vi "Main Page.vi"(8 "error in (no error)":errorcluster, 11 "Node Ptr":T1 format="%.0x") -> (0 "error out":errorcluster)   [LabVIEW 2019, in "UDP-Custom-Device System Explorer.lvlib"]
uses:
  UDP-Custom-Device System Explorer.lvlib
  <vilib>/NI VeriStand/Custom Device API/Custom Device Item Ref.ctl
  Types/Page References/Refs - Main Page.ctl
  <vilib>/NI VeriStand/Custom Device API/Custom Device API.lvlib
  <vilib>/NI VeriStand/Custom Device Tools/Custom Device Utility Library/Custom Device Utility Library.lvlib
  Property Accessors/Main Accessors.lvlib
panel:
  in  "Export Path":path
  in  "Export to File on Save":bool
  in  "Export Configuration Header":cluster{"Section Name":string}={"Section Name"="UDP Export Configuration Settings"}
  in  "Select Time-Stamp Channel":bool
  out "Timestamp Channel":string
  out "Version":string
  in  "SHDocVw.IWebBrowser":refnum<k7>(container)
  in  "Network Settings Header":cluster{"Section Name":string}={"Section Name"="UDP Settings"}
  in  "General Header":cluster{"Section Name":string}={"Section Name"="UDP Custom Device Information"}
  in  "Description":string
  in  "Name":string
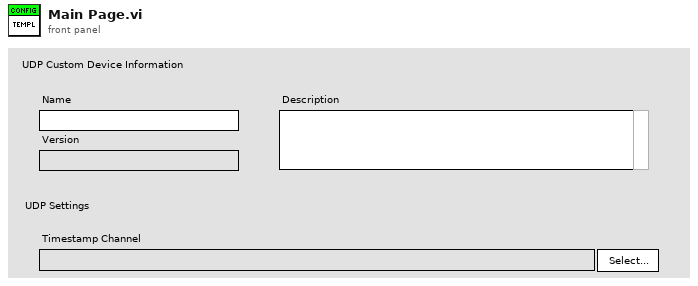
[diagram p1: front panel]
types:
  T1 = typedef "Custom Device API.lvlib/Custom Device Item Ref.ctl" = u64
  T2 = typedef "UDP-Custom-Device System Explorer.lvlib/Refs - Main Page.ctl" = cluster{"Name":refnum<vi>, "Timestamp Channel":refnum<vi>, "Export Path":refnum<vi>, "Export to File on Save":refnum<vi>}
  T3 = enum8{"Enabled", "Disabled", "Disabled and Grayed Out"}
  T4 = typedef "Custom Device API.lvlib/Custom Device Commands.ctl" = enum16{"Default", "Item renamed", "Shutdown", "Dynamic button pressed"}
  T5 = typedef "Custom Device API.lvlib/Custom Device Item Info.ctl" = cluster{"Name":string, "Is Channel":bool, "GUID":string, "Is Waveform":bool}
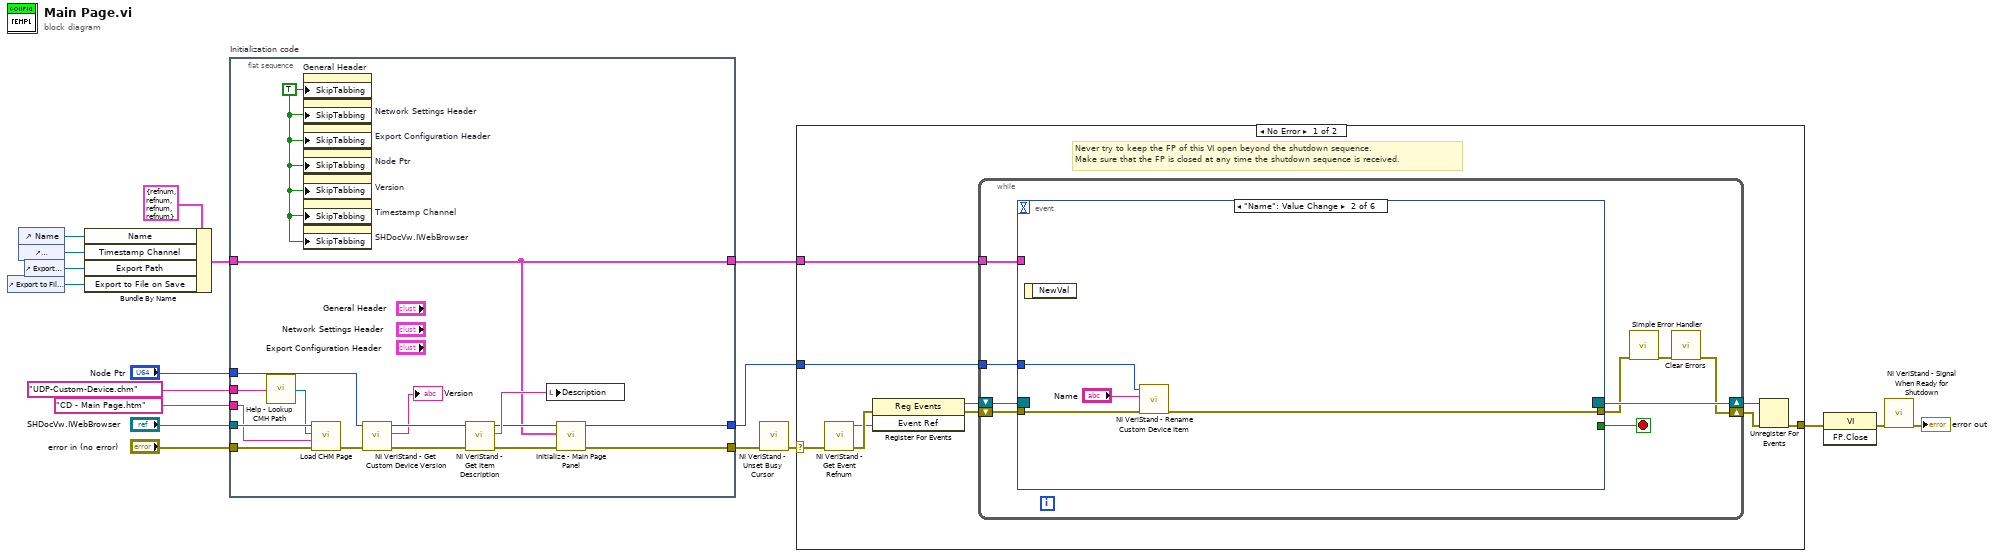
[diagram p0: block diagram]
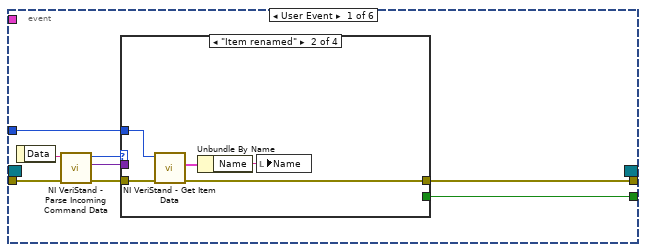
[diagram p2: hidden frame]
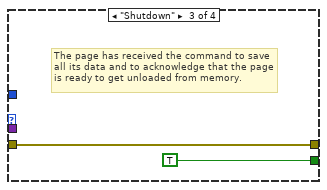
[diagram p4: hidden frame]
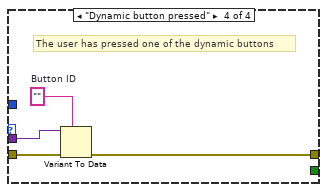
[diagram p5: hidden frame]
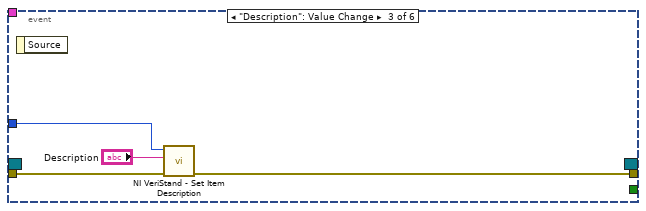
[diagram p6: hidden frame]
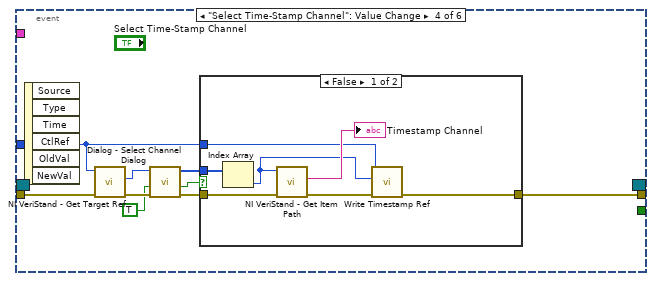
[diagram p7: hidden frame]
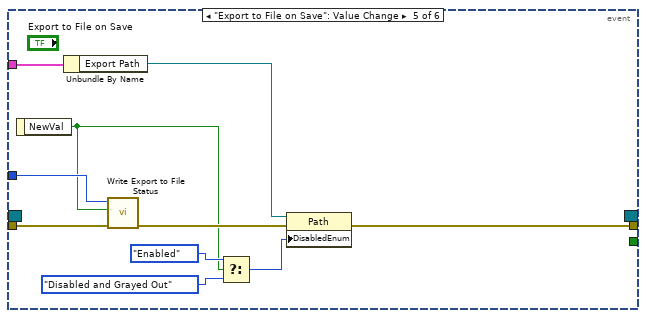
[diagram p9: hidden frame]
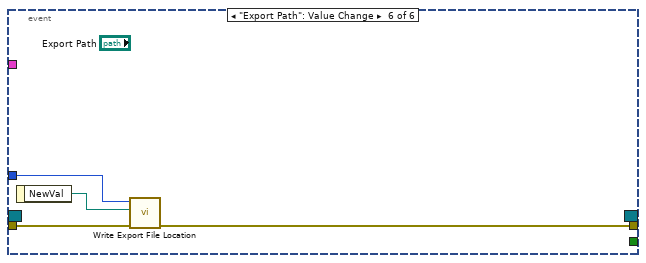
[diagram p10: hidden frame]
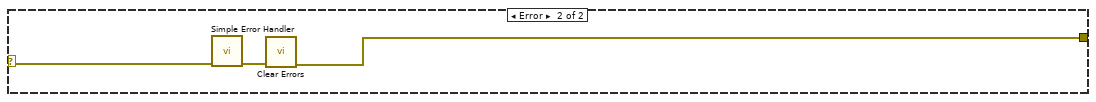
[diagram p11: hidden frame]
diagram:
  n1 = control-ref of="Export to File on Save"() -> (w4:refnum<vi>)
  n2 = control-ref of="Name"() -> (w1:refnum<vi>)
  n3 = control-ref of="Timestamp Channel"() -> (w6:refnum<vi>)
  n4 = control-ref of="Export Path"() -> (w5:refnum<vi>)
  n5 = Bundle By Name(cluster=T2 {"Name"=refnum, "Timestamp Channel"=refnum, "Export Path"=refnum, "Export to File on Save"=refnum} ("Main Page Refs"), "Name"=w1, "Timestamp Channel"=w6, "Export Path"=w5, "Export to File on Save"=w4) -> (w3:T2)
  n6 = flat-sequence "Initialization code" {
    tunnel: "error in (no error)" -> [w22]
    tunnel: "Node Ptr" -> [w35]
    tunnel: [w29] -> w14
    tunnel: [w28] -> w11
    tunnel: "SHDocVw.IWebBrowser" -> [w24]
    tunnel: "CD - Main Page.htm" ("HTML File") -> [w23]
    tunnel: "UDP-Custom-Device.chm" ("CD_CHM_FileName") -> [w21]
    tunnel: w3 -> [w26]
    tunnel: [w26] -> w2
    frame #0 {
      w19 = TRUE ("Skip When Tabbing")
      n7 = call "Help - Lookup CMH Path.vi"("Main CMH File"=w21) -> ("Compiled CMH Path"=w20:path)
      n8 = property on="General Header" class="Clust (strict)"("SkipTabbing"=w19) -> ()  [unwired: 2 in, 2 out]
      n9 = property on="Network Settings Header" class="Clust (strict)"("SkipTabbing"=w19) -> ()  [unwired: 2 in, 2 out]
      n10 = property on="Export Configuration Header" class="Clust (strict)"("SkipTabbing"=w19) -> ()  [unwired: 2 in, 2 out]
      n11 = property on="Node Ptr" class="DigNum (strict)"("SkipTabbing"=w19) -> ()  [unwired: 2 in, 2 out]
      n12 = property on="Version" class="Str"("SkipTabbing"=w19) -> ()  [unwired: 2 in, 2 out]
      n13 = property on="Timestamp Channel" class="Str"("SkipTabbing"=w19) -> ()  [unwired: 2 in, 2 out]
      n14 = property on="SHDocVw.IWebBrowser" class="AXCont"("SkipTabbing"=w19) -> ()  [unwired: 2 in, 2 out]
      n15 = call <vilib>:"Load CHM Page.vi"("error in (no error)"=w22, "HTML File"=w23, "Compiled CHM Path"=w20, "Web Browser Reference"=w24) -> ("error out"=w25:errorcluster)  [unwired: 7 in]
      n16 = call <vilib>:"NI VeriStand - Get Custom Device Version.vi"("error in (no error)"=w25, "Device Ref in"=w35) -> ("error out"=w34:errorcluster, "Value"=→"Version":string, "Device Ref out"=w33:T1)  [unwired: 7 in]
      n17 = call <vilib>:"NI VeriStand - Get Item Description.vi"("error in (no error)"=w34, "Item Ref in"=w33) -> ("error out"=w30:errorcluster, "Description"=w31:string, "Item Ref out"=w27:T1)  [unwired: 7 out]
      n18 = local write "Description"(w31) -> ()
      n19 = call "Initialize - Main Page Panel.vi"("error in (no error)"=w30, "Main Page References"=w26, "Item Ref in"=w27) -> ("error out"=w29:errorcluster, "Item Ref out"=w28:T1)  [unwired: 7 in]
    }
  }
  n20 = call <vilib>:"NI VeriStand - Unset Busy Cursor.vi"("error in (no error)"=w14) -> ("error out"=w13:errorcluster)  [unwired: 10 out]
  n21 = case shown="No Error" w13 {
    selector: w13 -> [w37 w116]
    tunnel: [w42 w114] -> w18
    tunnel: w11 -> [w38 _]
    tunnel: w2 -> [w36 _]
    frame No Error {
      # "Never try to keep the FP of this VI open beyond the shutdown sequence.\nMake sure that the FP is closed at any time the shutdown sequence is received."
      n22 = call <vilib>:"NI VeriStand - Get Event Refnum.vi"("error in (no error)"=w37) -> ("error out"=w45:errorcluster, "Event Ref"=w41:refnum<user-event>)  [unwired: 9 out]
      n23 = register-events(error in=w45, w41) -> (reference out=w39:refnum<event-registration>, error out=w40:errorcluster)  [unwired: 1 in]
      n24 = while {
        tunnel: w38 -> [w50]
        shift-right: [w47] -> w43
        shift-left: w40 -> [w53]
        shift-right: [w54] -> w44
        shift-left: w39 -> [w52]
        tunnel: w36 -> [w46]
        stop <- w51 stop-if-true
        n25 = event shown="[1] \"Name\": Value Change" {
          selector: w52 -> [_ _ _ _ _ _]
          dyn-events: [_ _ _ _ _ _] -> w54
          timeout: _ -> [_ _ _ _ _ _]
          tunnel: w53 -> [w62 w78 w81 w90 w102 w112]
          tunnel: [w58 _ _ _ _ _] -> w51
          tunnel: [w57 w77 w80 w91 w104 w111] -> w49
          tunnel: w50 -> [w56 w76 w82 w88 w103 w113]
          tunnel: w46 -> [_ _ _ _ w109 _]
          event User Event {
            n26 = event-data() -> ("Data"=w61:string)  [unwired: 1 out]
            n27 = call <vilib>:"NI VeriStand - Parse Incoming Command Data.vi"("error in (no error)"=w62, "Incoming data"=w61) -> ("error out"=w60:errorcluster, "Outgoing data"=w55:variant, "Action"=w59:T4)  [unwired: 7 out]
            n28 = case shown="\"Item renamed\"" w59 {
              tunnel: w60 -> [w63 w68 w69 w74]
              tunnel: [_ _ TRUE _] -> w58
              tunnel: [w63 w65 w69 w71] -> w57
              tunnel: w56 -> [_ w67 _ _]
              tunnel: w55 -> [_ _ _ w73]
              frame "Default", Default {
              }
              frame "Item renamed" {
                n29 = call <vilib>:"NI VeriStand - Get Item Data.vi"("error in (no error)"=w68, "Item Ref in"=w67) -> ("error out"=w65:errorcluster, "Item Info"=w66:T5)  [unwired: 8 out]
                n30 = Unbundle By Name(w66) -> ("Name"=w64:string)
                n31 = local write "Name"(w64) -> ()
              }
              frame "Shutdown" {
                # "The page has received the command to save all its data and to acknowledge that the page is ready to get unloaded from memory."
              }
              frame "Dynamic button pressed" {
                w72 = ""  # Button ID
                # "The user has pressed one of the dynamic buttons"
                n32 = Variant To Data(error in=w74, type=w72, Variant=w73) -> (error out=w71:errorcluster)  [unwired: 1 out]
              }
            }
          }
          event "Name": Value Change {
            n33 = event-data() -> ()  [unwired: 2 out]
            n34 = call <vilib>:"NI VeriStand - Rename Custom Device Item.vi"("error in (no error)"=w78, "New Name"="Name", "Item Ref in"=w76) -> ("error out"=w77:errorcluster)  [unwired: 1 in, 7 out]
          }
          event "Description": Value Change {
            n35 = event-data() -> ()  [unwired: 2 out]
            n36 = call <vilib>:"NI VeriStand - Set Item Description.vi"("error in (no error)"=w81, "Description"="Description", "Item Ref in"=w82) -> ("error out"=w80:errorcluster)  [unwired: 8 out]
          }
          event "Select Time-Stamp Channel": Value Change {
            n37 = event-data() -> ()  [unwired: 7 out]
            n38 = call <vilib>:"NI VeriStand - Get Target Ref.vi"("error in"=w90, "Item Ref in"=w88) -> ("error out"=w89:errorcluster, "Target Ref"=w87:T1)  [unwired: 6 in, 2 out]
            n39 = call "Dialog - Select Channel Dialog.vi"("error in (no error)"=w89, "Allow Section Selection (F)"=TRUE, "Root Item Ref"=w87) -> ("error out"=w85:errorcluster, "Canceled"=w83:bool, "Selected Channel Refs"=w84:T1[])  [unwired: 6 in]
            n40 = case shown="False" w83 {
              tunnel: [w92 w99] -> w91
              tunnel: w88 -> [w95 _]
              tunnel: w85 -> [w97 w99]
              tunnel: w84 -> [w98 _]
              frame False {
                n41 = Index Array(array=w98) -> (element=w94:T1)  [unwired: 1 in]
                n42 = call <vilib>:"NI VeriStand - Get Item Path.vi"("error in (no error)"=w97, "Item Ref in"=w94) -> ("error out"=w93:errorcluster, "Path"=→"Timestamp Channel":string)  [unwired: 6 in, 2 out]
                n43 = call "Write Timestamp Ref.vi"("error in (no error)"=w93, "Timestamp Ref"=w94, "Node Ptr"=w95) -> ("error out"=w92:errorcluster)  [unwired: 7 in, 1 out]
              }
              frame True {
              }
            }
          }
          event "Export to File on Save": Value Change {
            n44 = event-data() -> ("NewVal"=w100:bool)  [unwired: 1 out]
            n45 = Unbundle By Name(w109) -> ("Export Path"=w108:refnum<vi>)
            n46 = call "Write Export to File Status.vi"("error in (no error)"=w102, "Export to File Status"=w100, "Node Ptr"=w103) -> ("error out"=w101:errorcluster)  [unwired: 7 in, 1 out]
            n47 = Select(t=T3."Enabled" ("Disabled"), s=w100, f=T3."Disabled and Grayed Out" ("Disabled")) -> (s? t:f=w105:T3)
            n48 = property class="Path"(reference=w108, error in=w101, "DisabledEnum"=w105) -> (error out=w104:errorcluster)  [unwired: 1 out]
          }
          event "Export Path": Value Change {
            n49 = event-data() -> ("NewVal"=w110:path)  [unwired: 1 out]
            n50 = call "Write Export File Location.vi"("error in (no error)"=w112, "Export File Location"=w110, "Node Ptr"=w113) -> ("error out"=w111:errorcluster)  [unwired: 7 in, 1 out]
          }
        }
        n51 = call <vilib>:"Simple Error Handler.vi"("error in (no error)"=w49) -> ("error out"=w48:errorcluster)  [unwired: 1 in, 7 out]
        n52 = call <vilib>:"Clear Errors.vi"("error in (no error)"=w48) -> ("error out"=w47:errorcluster)  [unwired: 1 in, 5 out]
      }
      n53 = Unregister For Events(event registration refnum=w44, error in=w43) -> (error out=w42:errorcluster)
    }
    frame Error {
      n54 = call <vilib>:"Simple Error Handler.vi"("error in (no error)"=w116) -> ("error out"=w115:errorcluster)  [unwired: 1 in, 7 out]
      n55 = call <vilib>:"Clear Errors.vi"("error in (no error)"=w115) -> ("error out"=w114:errorcluster)  [unwired: 1 in, 5 out]
    }
  }
  n56 = invoke class="VI" method="FP.Close"(error in=w18) -> (error out=w17:errorcluster)  [unwired: 2 in, 2 out]
  n57 = call <vilib>:"NI VeriStand - Signal When Ready for Shutdown.vi"("error in (no error)"=w17) -> ("error out"=→"error out":errorcluster)  [unwired: 10 out]
